vi "XYZCWaveforms.vi"(3 "Microscope Settings":T1={"Mode"=enum."X", "Slit"={"Scanning Mode"=0.0, "Slit Width /%"=0.0}, "Colour"=[], "Exposure/ms"=0.0, "Piezo Position /um"=0.0, "ROI"={"X"={"Start /px"=0.0, "Step /px"=0.0, "Range /px"=0.0}, "Y"={"Start /px"=0.0, "Step /px"=0.0, "Range /px"=0.0}, "Z "={"Start /um"=0.0, "Step/um"=0.0, "Range /um"=0.0}, "T "={"Start /s"=0.0, "Step /s"=0.0, "Range /s"=0.0}}, "Samples per millisecond"=0.0, "Relax/ms"=0.0, "Readout Direction"=0.0, "Trigger Source"=0.0, "Camera Delay /ms"=0.0, "Under Scan /ms"=0.0, "Waveforms"={"Analogue Out"=[], "Digital Out"=[]}} {"Under Scan /ms" min=0.0 max=10.0 step=0.05; "ROI"."T"."Range /s" min=0.0 max=10.0 step=0.05; "ROI"."T"."Step /s" min=0.0 max=10.0 step=0.05; "ROI"."T"."Start /s" min=0.0 max=10.0 step=0.05; "ROI"."X"."Range /px" min=0.0 max=10.0 step=0.05; "ROI"."X"."Step /px" min=0.0 max=10.0 step=0.05; "ROI"."X"."Start /px" min=0.0 max=10.0 step=0.05; "ROI"."Y"."Range /px" min=0.0 max=10.0 step=0.05; "ROI"."Y"."Step /px" min=0.0 max=10.0 step=0.05; "ROI"."Y"."Start /px" min=0.0 max=10.0 step=0.05; "ROI"."Z"."Range /um" min=0.0 max=10.0 step=0.05; "ROI"."Z"."Step/um" min=0.0 max=10.0 step=0.05; "ROI"."Z"."Start /um" min=0.0 max=10.0 step=0.05; "Colour"."Colour"."Filter" items=["Empty"=1, ""=2, ""=3, "561"=4, ""=5, "488"=6]; "Camera Delay /ms" min=0.0 max=10.0 step=0.05; "Trigger Source" items=["Internal"=1.0, "External"=2.0]; "Readout Direction" items=["Forward"=1.0, "Backward"=2.0]; "Slit"."Scanning Mode" items=["Full Frame"=1.0, "Slit Scanning"=12.0]; "Piezo Position /um" min=0.0 max=10.0 step=0.05}) -> (0 "Array":digitalwaveform[](array[waveform]), 1 "Analogue Out out":waveform(dbl)[](array[waveform]))   [LabVIEW 2016]
uses:
  controls/Microscope Settings.ctl
  controls/ColourCalibration.ctl
  <vilib>/Waveform/WDTOps.llb/WDT Append Waveforms DBL.vi
  <vilib>/Waveform/DWDTOps.llb/DWDT Append Digital Samples.vi
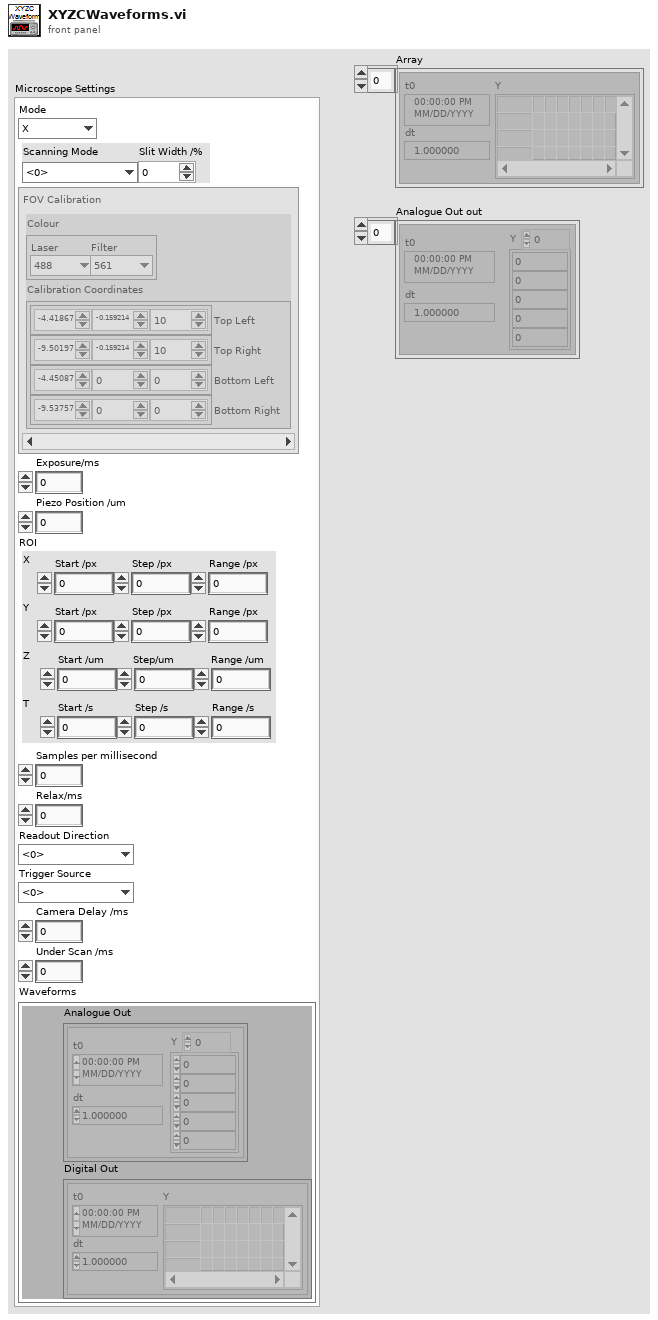
[diagram p1: front panel]
types:
  T1 = typedef "Microscope Settings.ctl" = cluster{"Mode":enum16{"Brightfield", "X", "XY", "XYZ", "XYZT", "XYZC", "Tweezers", "Virus"}, "Slit":cluster{"Scanning Mode":dbl, "Slit Width /%":dbl}, "Colour":T2, "Exposure/ms":dbl, "Piezo Position /um":dbl, "ROI":cluster{"X":cluster{"Start /px":dbl, "Step /px":dbl, "Range /px":dbl}, "Y":cluster{"Start /px":dbl, "Step /px":dbl, "Range /px":dbl}, "Z ":cluster{"Start /um":dbl, "Step/um":dbl, "Range /um":dbl}, "T ":cluster{"Start /s":dbl, "Step /s":dbl, "Range /s":dbl}}, "Samples per millisecond":dbl, "Relax/ms":dbl, "Readout Direction":dbl, "Trigger Source":dbl, "Camera Delay /ms":dbl, "Under Scan /ms":dbl, "Waveforms":cluster{"Analogue Out":waveform(dbl)[], "Digital Out":digitalwaveform[]}}
  T2 = typedef "ColourCalibration.ctl" = cluster{"Colour":cluster{"Laser":enum16{"Brightfield", "445", "488", "561", "647"}, "Filter":u16}, "Calibration Coordinates":cluster{"Top Left":dbl[], "Top Right":dbl[], "Bottom Left":dbl[], "Bottom Right":dbl[]}}[]
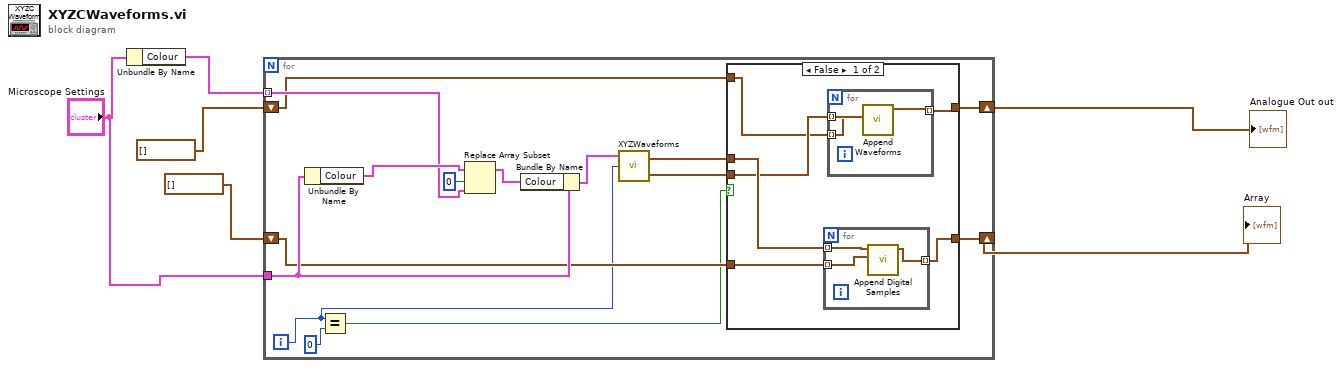
[diagram p0: block diagram]
diagram:
  n1 = Unbundle By Name("Microscope Settings") -> ("Colour"=w6:T2)
  n2 = for {
    tunnel: "Microscope Settings" -> [w17]
    tunnel: w6 -> [w19] mode=indexing
    shift-right: [w14] -> w4
    shift-left: digitalwaveform[] [] ("Digital Out") -> [w13]
    shift-right: [w11] -> w3
    shift-left: waveform(dbl)[] [] ("Analogue Out") -> [w10]
    i -> [w7]
    n3 = Unbundle By Name(w17) -> ("Colour"=w21:T2)
    n4 = Equal?(x=w7, y=0) -> (x = y?=w8:bool)
    n5 = Replace Array Subset(array=w21, new element=w19, index=0) -> (w18:T2)
    n6 = Bundle By Name(cluster=w17, "Colour"=w18) -> (w16:T1)
    n7 = call "XYZWaveforms.vi"("Colour Channel"=w7, "Microscope Settings"=w16) -> ("Analogue Out out"=w12:waveform(dbl)[], "Digital Out out"=w15:digitalwaveform[])  [unwired: 1 in]
    n8 = case shown="False" w8 {
      tunnel: w15 -> [w27 w34]
      tunnel: [w26 w34] -> w14
      tunnel: w13 -> [w25 _]
      tunnel: w12 -> [w24 w35]
      tunnel: [w23 w35] -> w11
      tunnel: w10 -> [w22 _]
      frame False {
        n9 = for {
          tunnel: w25 -> [w32] mode=indexing
          tunnel: w27 -> [w33] mode=indexing
          tunnel: [w31] -> w26 mode=indexing
          n10 = call-poly <vilib>:"Append Digital Samples.vi"("digital waveform B"=w32, "digital waveform A"=w33) -> ("digital waveform out"=w31:digitalwaveform)  [unwired: 8 in, 1 out]
        }
        n11 = for {
          tunnel: w22 -> [w29] mode=indexing
          tunnel: w24 -> [w30] mode=indexing
          tunnel: [w28] -> w23 mode=indexing
          n12 = call-poly <vilib>:"Append Waveforms.vi"("waveform B"=w29, "waveform A"=w30) -> ("waveform out"=w28:waveform(dbl))  [unwired: 8 in, 1 out]
        }
      }
      frame True {
      }
    }
  }
  "Array" <- w4
  "Analogue Out out" <- w3
